vi "SrsQcm200FandRandM.vi"(0 "VISA in":refnum<visa-resource-name>="GPIB0::3::INSTR", 1 "Reference time in":u32, 11 "error in (no error)":errorcluster) -> (4 "VISA out":refnum<visa-resource-name>, 6 "Frequency out":dbl format="%.6e", 8 "timestamp out":dbl format="%.2f", 10 "Resistance out":dbl format="%.6e", 13 "F vs T out":T2 {"Frequency out" format="%.2f"; "timestamp out" format="%.2f"}, 14 "R vs T out":T1 {"Resistance out" format="%.2f"; "timestamp out" format="%.2f"}, 15 "error out":errorcluster)   [LabVIEW 2013]
doc: "This VI returns the QCM200 frequency and resistance values together.\n\nCopyright 2004 Stanford Research Systems"
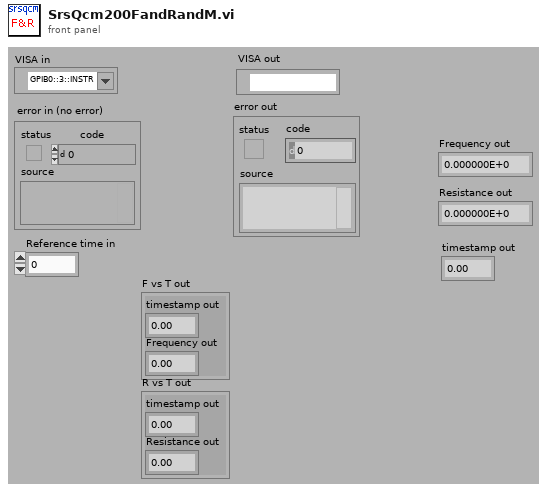
[diagram p1: front panel]
types:
  T1 = cluster{"timestamp out":dbl, "Resistance out":dbl}
  T2 = cluster{"timestamp out":dbl, "Frequency out":dbl}
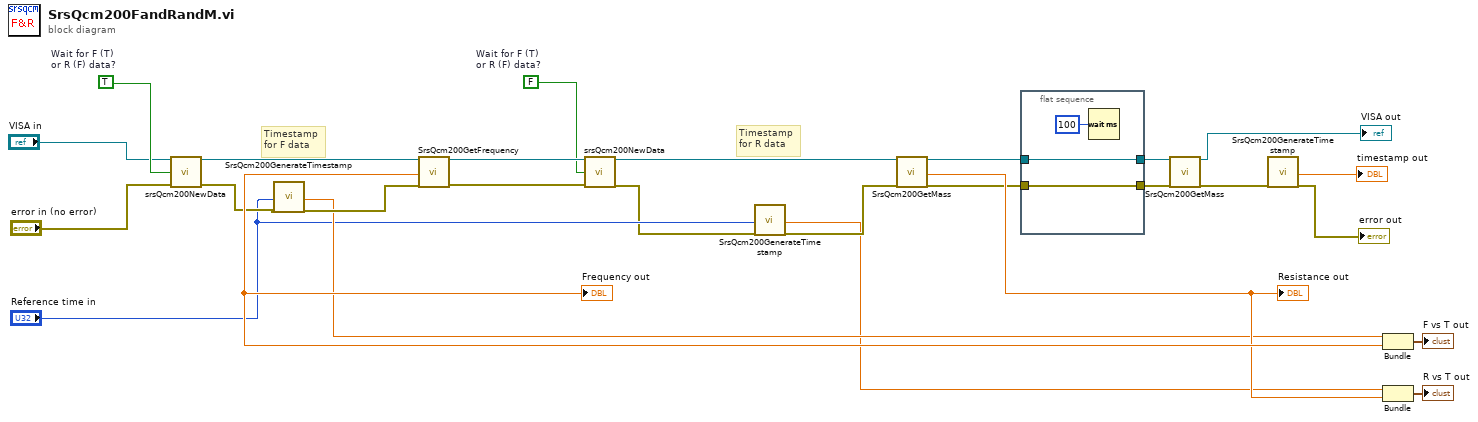
[diagram p0: block diagram]
diagram:
  w24 = FALSE  # Wait for F (T) or R (F) data?
  w23 = TRUE  # Wait for F (T) or R (F) data?
  # "Timestamp\nfor R data"
  # "Timestamp\nfor F data"
  n1 = call <instrlib>:"srsQcm200NewData.vi"("VISA in"="VISA in", "Wait for F (T)\nor R (F) data?"=w23, "error in (no error)"="error in (no error)") -> ("VISA out"=w27:refnum<visa-resource-name>, "error out"=w14:errorcluster)  [unwired: 11 in]
  n2 = call <instrlib>:"SrsQcm200GenerateTimestamp.vi"("Reference time in"="Reference time in", "Error In"=w14) -> ("timestamp out"=w11:dbl, "error out"=w13:errorcluster)  [unwired: 16 in]
  n3 = call <instrlib>:"SrsQcm200GetFrequency.vi"("VISA in"=w27, "error in (no error)"=w13) -> ("VISA out"=w25:refnum<visa-resource-name>, "Frequency out"=w18:dbl, "error out"=w26:errorcluster)  [unwired: 15 in]
  "Frequency out" <- w18
  n4 = call <instrlib>:"srsQcm200NewData.vi"("VISA in"=w25, "Wait for F (T)\nor R (F) data?"=w24, "error in (no error)"=w26) -> ("VISA out"=w20:refnum<visa-resource-name>, "error out"=w9:errorcluster)  [unwired: 11 in]
  n5 = call <instrlib>:"SrsQcm200GenerateTimestamp.vi"("Reference time in"="Reference time in", "Error In"=w9) -> ("timestamp out"=w7:dbl, "error out"=w8:errorcluster)  [unwired: 16 in]
  n6 = call "SrsQcm200GetMass.vi"("VISA in"=w20, "error in (no error)"=w8) -> ("VISA out"=w6:refnum<visa-resource-name>, "Resistance out"=w16:dbl, "error out"=w5:errorcluster)  [unwired: 15 in]
  "Resistance out" <- w16
  n7 = flat-sequence {
    tunnel: w6 -> [w30]
    tunnel: w5 -> [w29]
    tunnel: [w30] -> w3
    tunnel: [w29] -> w2
    frame #0 {
      n8 = Wait (ms)(milliseconds to wait=u32 100) -> ()  [unwired: 1 out]
    }
  }
  n9 = call "SrsQcm200GetMass.vi"("VISA in"=w3, "error in (no error)"=w2) -> ("VISA out"=→"VISA out":refnum<visa-resource-name>, "error out"=w4:errorcluster)  [unwired: 15 in, 1 out]
  n10 = call <instrlib>:"SrsQcm200GenerateTimestamp.vi"("Error In"=w4) -> ("timestamp out"=→"timestamp out":dbl, "error out"=→"error out":errorcluster)  [unwired: 17 in]
  n11 = Bundle("timestamp out"=w11, "Frequency out"=w18) -> (→"F vs T out":T2)  [unwired: 1 in]
  n12 = Bundle("timestamp out"=w7, "Resistance out"=w16) -> (→"R vs T out":T1)  [unwired: 1 in]
